vi "Correction.vi"(0 "Calibrated Image":T1, 5 "Search Direction":enum16{"Horizontal", "Vertical"}(ring), 7 "AvgMinMax":enum16{"Average", "Max", "Min", "Max2"}(ring), 9 "appended array":cluster{"X":sgl, "Y":sgl}[][](array[cluster]), 11 "error in (no error)":errorcluster) -> (4 "Mesurement Value":sgl, 15 "error IO":errorcluster)   [LabVIEW 2014]
uses:
  <vilib>/vision/Image Controls.llb/IMAQ Image.ctl
  <vilib>/vision/NI_Vision_Development_Module.lvlib
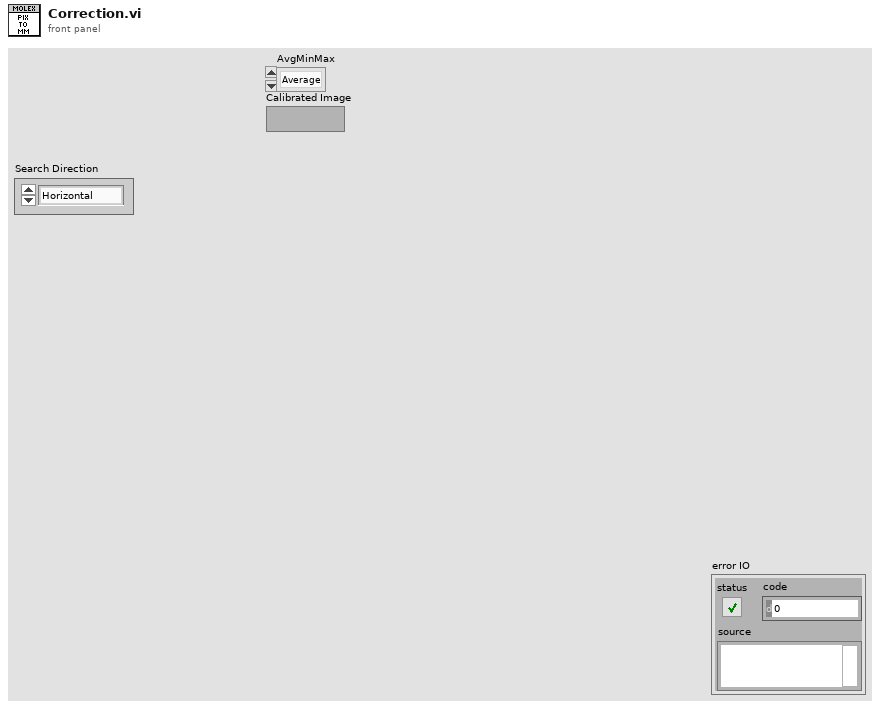
[diagram p1: front panel]
types:
  T1 = typedef "IMAQ Image.ctl" = refnum<image>
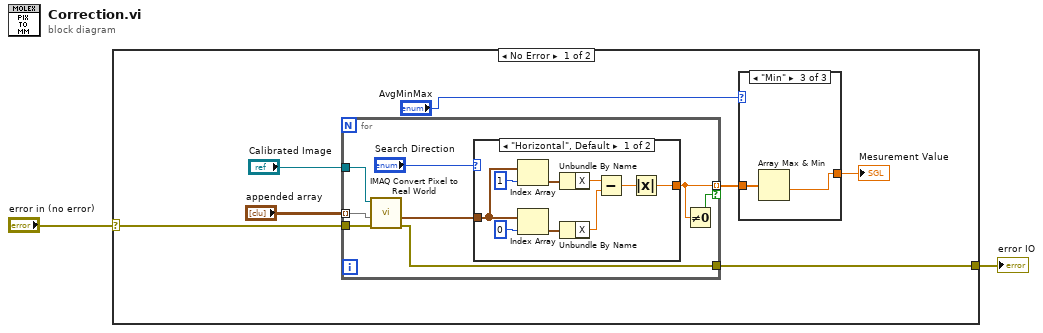
[diagram p0: block diagram]
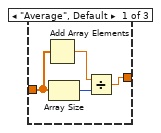
[diagram p2: hidden frame]
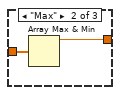
[diagram p3: hidden frame]
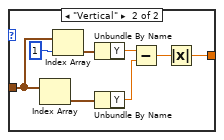
[diagram p4: hidden frame]
diagram:
  n1 = case shown="No Error" "error in (no error)" {
    selector: "error in (no error)" -> [w6 w43]
    tunnel: [w5 w43] -> w1
    frame No Error {
      n2 = for {
        tunnel: "appended array" -> [w25] mode=indexing
        tunnel: "Calibrated Image" -> [w24]
        tunnel: [w18] -> w8 mode=indexing if=w19
        tunnel: w6 -> [w21]
        tunnel: [w20] -> w5
        n3 = call "IMAQ Convert Pixel to Real World"("error in (no error)"=w21, "Array of Pixel Coordinates"=w25, "Calibrated Image"=w24) -> ("error out"=w20:errorcluster, "Array of Real World Coordinates"=w23:cluster{"X":sgl, "Y":sgl}[])  [unwired: 3 in, 4 out]
        n4 = case shown="\"Horizontal\", Default" "Search Direction" {
          tunnel: w23 -> [w29 w42]
          tunnel: [w26 w35] -> w18
          frame "Horizontal", Default {
            n5 = Index Array(array=w29, index=1) -> (element=w31:cluster{"X":sgl, "Y":sgl})
            n6 = Index Array(array=w29, index=0) -> (element=w33:cluster{"X":sgl, "Y":sgl})
            n7 = Unbundle By Name(w31) -> ("X"=w30:sgl)
            n8 = Unbundle By Name(w33) -> ("X"=w32:sgl)
            n9 = Subtract(x=w30, y=w32) -> (x-y=w28:sgl)
            n10 = Absolute Value(x=w28) -> (abs(x)=w26:sgl)
          }
          frame "Vertical" {
            n11 = Index Array(array=w42) -> (element=w41:cluster{"X":sgl, "Y":sgl})  [unwired: 1 in]
            n12 = Index Array(array=w42, index=1) -> (element=w39:cluster{"X":sgl, "Y":sgl})
            n13 = Unbundle By Name(w39) -> ("Y"=w38:sgl)
            n14 = Unbundle By Name(w41) -> ("Y"=w40:sgl)
            n15 = Subtract(x=w38, y=w40) -> (x-y=w36:sgl)
            n16 = Absolute Value(x=w36) -> (abs(x)=w35:sgl)
          }
        }
        n17 = Not Equal To 0?(x=w18) -> (x != 0?=w19:bool)
      }
      n18 = case shown="\"Min\"" "AvgMinMax" {
        tunnel: w8 -> [w13 w15 w17]
        tunnel: [w10 w14 w16] -> w7
        frame "Average", Default {
          n19 = Add Array Elements(numeric array=w13) -> (sum=w12:sgl)
          n20 = Array Size(array=w13) -> (size(s)=w11:i32)
          n21 = Divide(x=w12, y=w11) -> (x/y=w10:sgl)
        }
        frame "Max" {
          n22 = Array Max & Min(array=w15) -> (max value=w14:sgl)  [unwired: 3 out]
        }
        frame "Min" {
          n23 = Array Max & Min(array=w17) -> (min value=w16:sgl)  [unwired: 3 out]
        }
      }
      "Mesurement Value" <- w7
    }
    frame Error {
    }
  }
  "error IO" <- w1
